vi "FestoCPX.statusExtract.vi"(1 "Status byte":u8 format="%.0x") -> (0 "Status":T1)   [LabVIEW 2013]
uses:
  FestoCPX.status.ctl
panel:
  # "out"
  # "in"
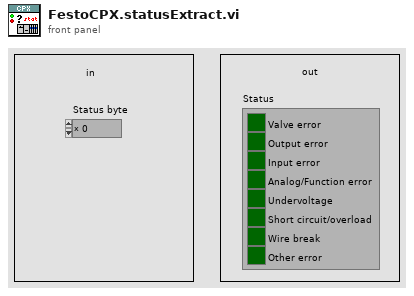
[diagram p1: front panel]
types:
  T1 = typedef "FestoCPX.status.ctl" = cluster{"Valve error":bool, "Output error":bool, "Input error":bool, "Analog/Function error":bool, "Undervoltage":bool, "Short circuit/overload":bool, "Wire break":bool, "Other error":bool}
  T2 = cluster{"Boolean array[0]":bool, "Boolean array[1]":bool, "Boolean array[2]":bool, "Boolean array[3]":bool, "Boolean array[4]":bool, "Boolean array[5]":bool, "Boolean array[6]":bool, "Boolean array[7]":bool}
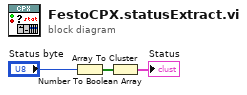
[diagram p0: block diagram]
diagram:
  n1 = Number To Boolean Array(number="Status byte") -> (Boolean array=w2:bool[])
  n2 = Array To Cluster(array=w2) -> (cluster=→"Status":T2)
